vi "Mindsensors TouchMux Config.vi"(10 "Node Data":T1, 11 "NXT":T2) -> ()   [LabVIEW 2010]
uses:
  <vilib>/NXT/Subs/LVHSConnector.ctl
  Datatypes/Node.ctl
  UI Controls/PlugInControls/Pluginbackground.ctl
  <vilib>/Utility/miscctls.llb/LVPointTypeDef.ctl
  <vilib>/NXT/Block Support/HWPage.SensorType.ctl
  <vilib>/NXT/Block Support/HWPage.SensorMode.ctl
  ConvertNodeAddrSensor.vi
panel:
  out "TouchMux 3":bool
  out "TouchMux 2":bool
  out "TouchMux 1":bool
  in  "Output":string
  out "?":dbl format="%#.2g"
  out "number":i8
  in  "NXT Port":string
  in  "Name":string
  out "Headline":string="Type (auto populated)"
  in  "Sensor Parameters":string
  in  "Instance Specific Data":cluster{"Example Data":dbl}
  in  "Reset":bool
  in  "Save":bool
  in  "Stop":bool
  out "Background":T3=TRUE
  # "<- No controls below this line"
  # "Common controls such as Buttons, Rings, Sliders, Graphs, Decorations, etc can be found in the <labview>\\Targets\\NI\\NXT\\NXT Toolkit\\Schematic Editor\\UI Controls\\Plugin Controls\\ folder. Use these controls when possible to ensure a consistent look and feel with LabVIEW Education Edition."
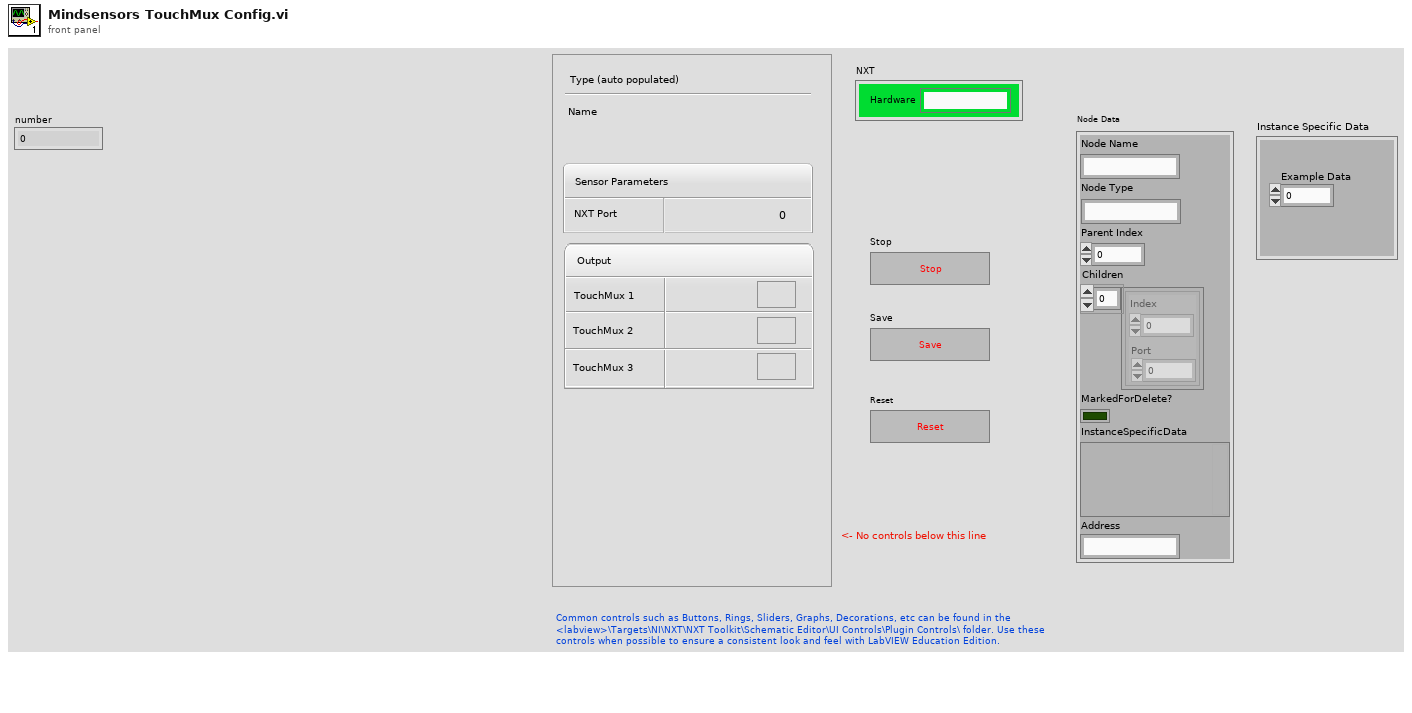
[diagram p1: front panel]
types:
  T1 = typedef "Node.ctl" = cluster{"Node Name":string, "Node Type":string, "Parent Index":i16, "Children":cluster{"Index":u16, "Port":u16}[], "MarkedForDelete?":bool, "InstanceSpecificData":variant, "Address":string}
  T2 = typedef "LVHSConnector.ctl" = cluster{"Hardware":string, "Flattened String":string}
  T3 = typedef "Pluginbackground.ctl" = bool
  T4 = typedef "LVPointTypeDef.ctl" = cluster{"Horizontal":i16, "Vertical":i16}
  T5 = typedef "HWPage.SensorType.ctl" = u8
  T6 = typedef "HWPage.SensorMode.ctl" = u8
  T7 = enum8{"Enabled", "Disabled", "Disabled and Grayed Out"}
  T8 = typedef "NXT_InputPort.ctl" = u8
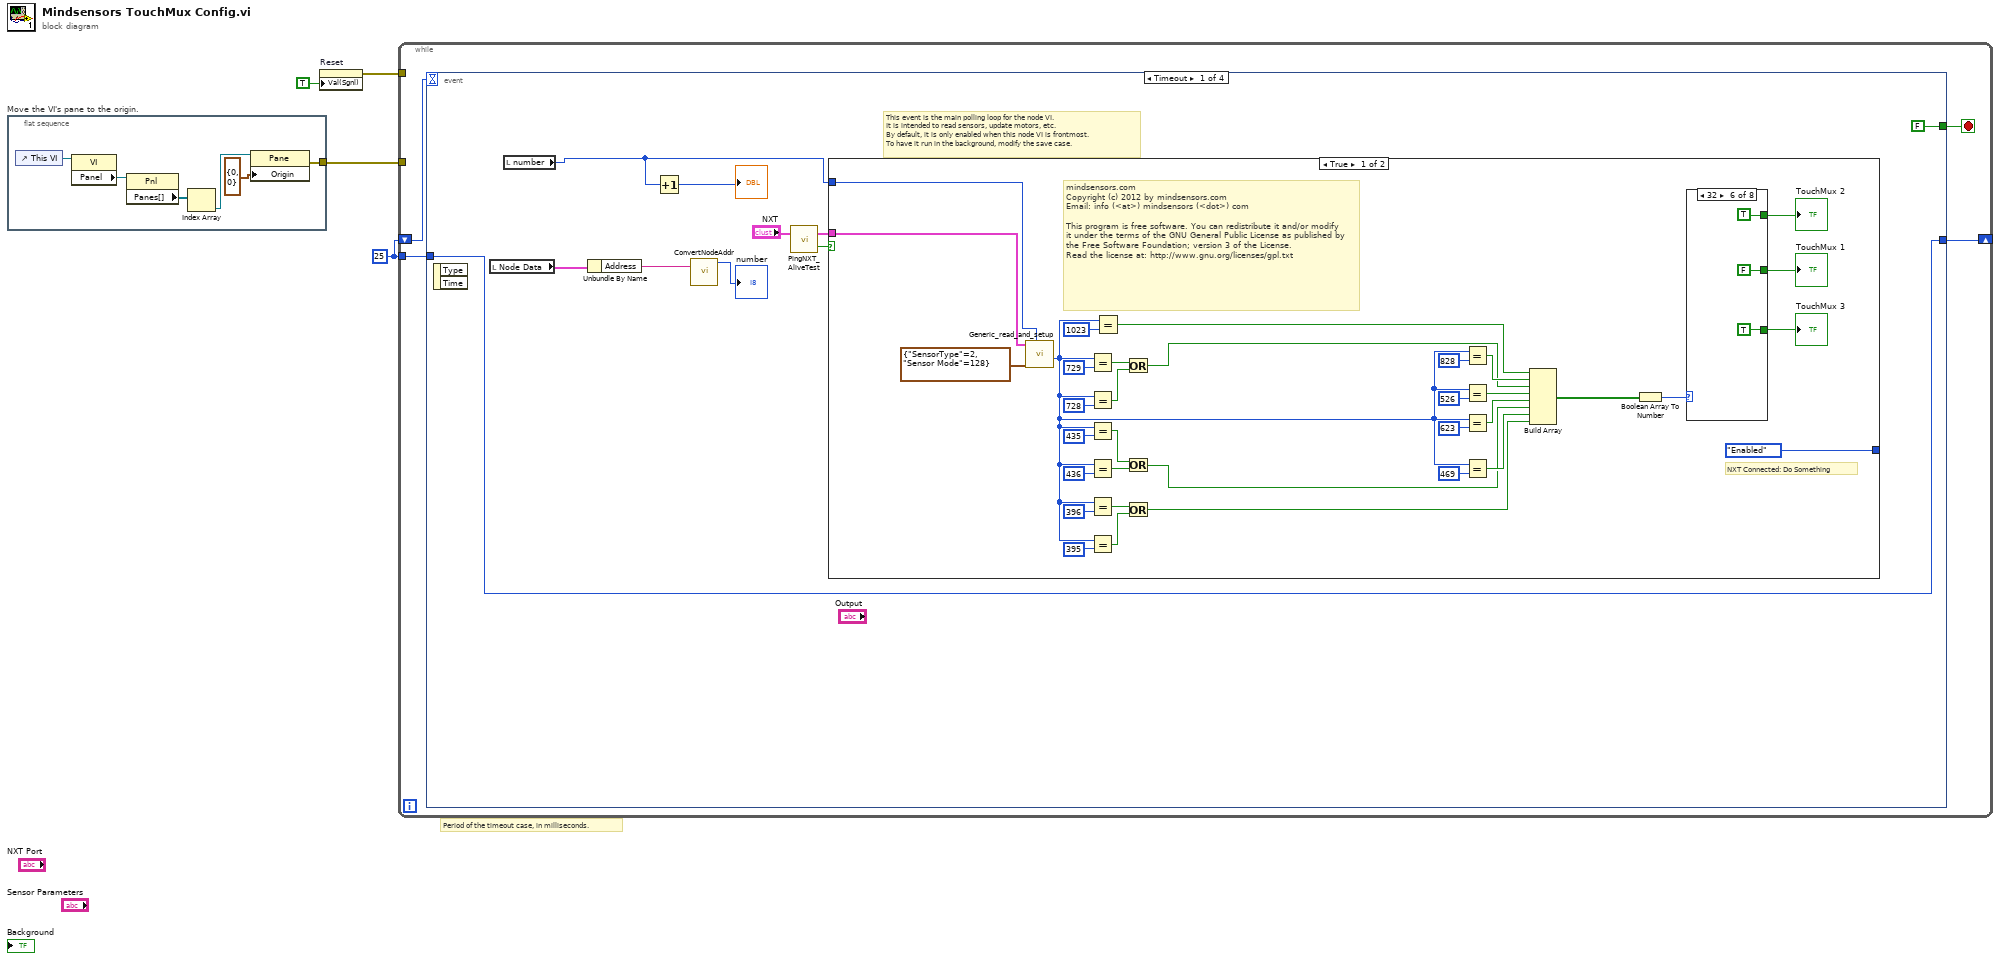
[diagram p0: block diagram]
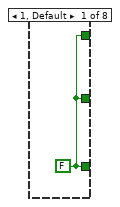
[diagram p2: hidden frame]
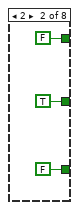
[diagram p3: hidden frame]
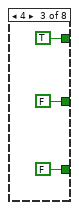
[diagram p4: hidden frame]
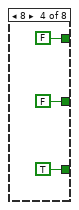
[diagram p5: hidden frame]
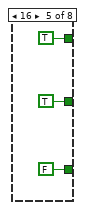
[diagram p6: hidden frame]
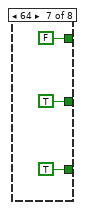
[diagram p7: hidden frame]
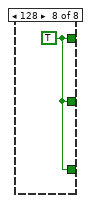
[diagram p8: hidden frame]
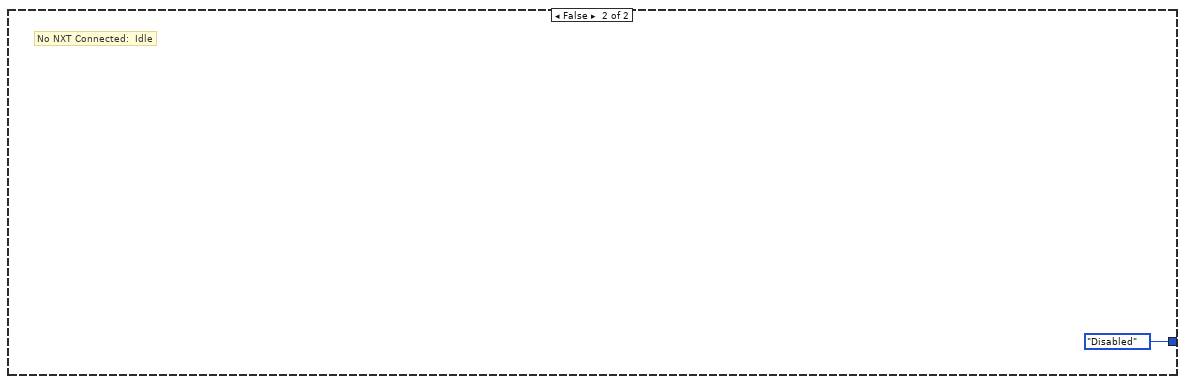
[diagram p9: hidden frame]
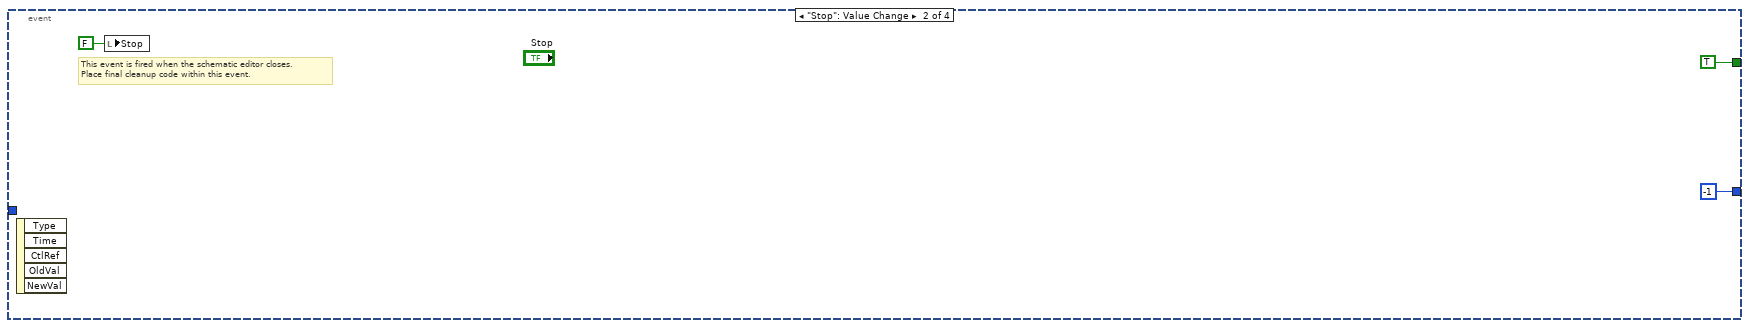
[diagram p10: hidden frame]
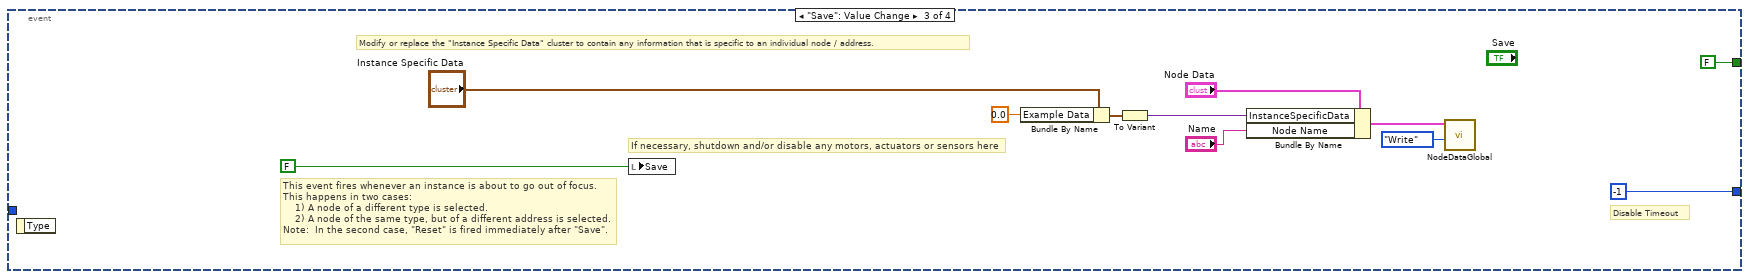
[diagram p11: hidden frame]
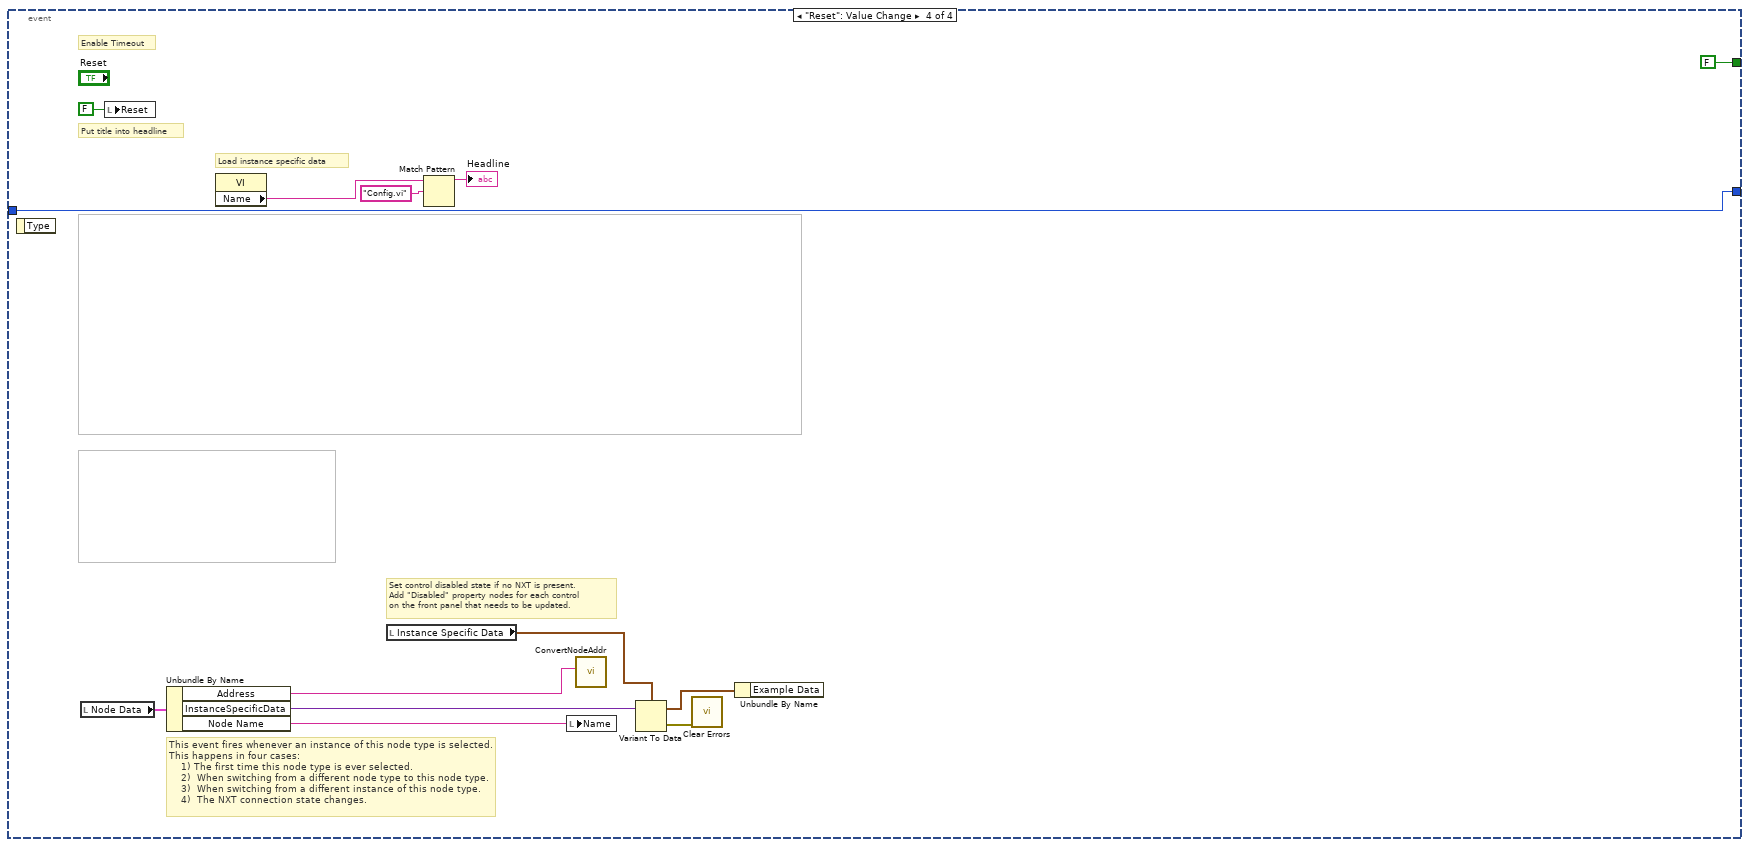
[diagram p12: hidden frame]
diagram:
  w2 = 25
  # "Period of the timeout case, in milliseconds."
  n1 = flat-sequence "Move the VI's pane to the origin." {
    tunnel: [w5] -> w1
    frame #0 {
      n2 = control-ref of="This VI"() -> (w6:refnum<vi>)
      n3 = property class="VI"(reference=w6) -> ("Panel"=w7:refnum<vi>)  [unwired: 1 in, 2 out]
      n4 = property class="Pnl"(reference=w7) -> ("Panes[]"=w8:refnum<vi>[])  [unwired: 1 in, 2 out]
      n5 = Index Array(array=w8) -> (element=w9:refnum<vi>)  [unwired: 1 in]
      n6 = property class="Pane"(reference=w9, "Origin"=T4 {"Horizontal"=0, "Vertical"=0}) -> (error out=w5:errorcluster)  [unwired: 1 in, 1 out]
    }
  }
  n7 = property on="Reset" class="Bool (strict)"("Val(Sgnl)"=TRUE ("Value (Signaling)")) -> (error out=w3:errorcluster)  [unwired: 2 in, 1 out]
  n8 = while {
    tunnel: w3 -> [_]
    shift-right: [w12] -> _
    shift-left: w2 -> [w13]
    tunnel: w2 -> [w11]
    tunnel: w1 -> [_]
    stop <- w14 stop-if-true
    n9 = event shown="[0] Timeout" {
      selector: _ -> [_ _ _ _]
      dyn-events: _ -> [_ _ _ _]
      timeout: w13 -> [_ _ _ _]
      tunnel: [FALSE TRUE FALSE FALSE] -> w14
      tunnel: [w23 -1 -1 w103] -> w12
      tunnel: w11 -> [w23 _ _ w103]
      event Timeout {
        # "This event is the main polling loop for the node VI.\nIt is intended to read sensors, update motors, etc.\nBy default, it is only enabled when this node VI is frontmost.\nTo have it run in the background, modify the save case."
        n10 = event-data() -> ()  [unwired: 1 in, 2 out]
        n11 = local read "Node Data"() -> (w21:T1)
        n12 = local read "number"() -> (w16:i8)
        n13 = Unbundle By Name(w21) -> ("Address"=w18:string)
        n14 = Increment(x=w16) -> (x+1=→"?":i8)
        n15 = call-poly "ConvertNodeAddr.vi"("Sensor Port"=w18) -> ("NXT Port"=→"number":T8)  [unwired: 6 in, 4 out]
        n16 = call <vilib>:"PingNXT_AliveTest.vi"("NXT"="NXT") -> ("connected?"=w20:bool, "NXT"=w19:T2)  [unwired: 1 in]
        n17 = case shown="True" w20 {
          tunnel: [T7."Enabled" ("Disabled") T7."Disabled" ("Disabled")] -> _
          tunnel: w19 -> [w57 _]
          tunnel: w16 -> [w58 _]
          frame True {
            # "mindsensors.com\nCopyright (c) 2012 by mindsensors.com\nEmail: info (<at>) mindsensors (<dot>) com\n\nThis program is free software. You can redistribute it and/or modify\nit under the terms of the GNU General Public License as published by\nthe Free Software Foundation; version 3 of the License.\nRead the license at: http://www.gnu.org/licenses/gpl.txt"
            # "NXT Connected: Do Something"
            n18 = call <vilib>:"Generic_read_and_setup.vi"("Port"=w58, "Sensor Setup"=cluster{"SensorType":T5, "Sensor Mode":T6} {"SensorType"=2, "Sensor Mode"=128}, "NXT In"=w57) -> ("Raw"=w28:u16)  [unwired: 6 in, 2 out]
            n19 = Equal?(x=w28, y=u16 729) -> (x = y?=w37:bool)
            n20 = Equal?(x=w28, y=u16 728) -> (x = y?=w35:bool)
            n21 = Equal?(x=w28, y=u16 435) -> (x = y?=w32:bool)
            n22 = Equal?(x=w28, y=u16 436) -> (x = y?=w31:bool)
            n23 = Equal?(x=w28, y=u16 396) -> (x = y?=w26:bool)
            n24 = Equal?(x=w28, y=u16 395) -> (x = y?=w27:bool)
            n25 = Equal?(x=w28, y=1023) -> (x = y?=w52:bool)
            n26 = Or(x=w37, y=w35) -> (x .or. y?=w34:bool)
            n27 = Or(x=w32, y=w31) -> (x .or. y?=w30:bool)
            n28 = Or(x=w26, y=w27) -> (x .or. y?=w25:bool)
            n29 = Equal?(x=w28, y=u16 828) -> (x = y?=w51:bool)
            n30 = Equal?(x=w28, y=u16 526) -> (x = y?=w50:bool)
            n31 = Equal?(x=w28, y=u16 623) -> (x = y?=w42:bool)
            n32 = Equal?(x=w28, y=u16 469) -> (x = y?=w41:bool)
            n33 = Build Array(w52, w51, w34, w50, w42, w30, w41, w25) -> (w55:bool[])
            n34 = Boolean Array To Number(Boolean array=w55) -> (number=w54:u32)
            n35 = case shown="32" w54 {
              tunnel: [w60 FALSE ("TouchMux 3") FALSE ("TouchMux 3") TRUE ("TouchMux 3") FALSE ("TouchMux 3") TRUE ("TouchMux 3") TRUE ("TouchMux 3") w79] -> w40
              tunnel: [w60 FALSE ("TouchMux 3") TRUE ("TouchMux 3") FALSE ("TouchMux 3") TRUE ("TouchMux 3") TRUE ("TouchMux 3") FALSE ("TouchMux 3") w79] -> w39
              tunnel: [w60 TRUE ("TouchMux 3") FALSE ("TouchMux 3") FALSE ("TouchMux 3") TRUE ("TouchMux 3") FALSE ("TouchMux 3") TRUE ("TouchMux 3") w79] -> w38
              frame 1, Default {
                w60 = FALSE ("TouchMux 3")
              }
              frame 2 {
              }
              frame 4 {
              }
              frame 8 {
              }
              frame 16 {
              }
              frame 32 {
              }
              frame 64 {
              }
              frame 128 {
                w79 = TRUE ("TouchMux 3")
              }
            }
            "TouchMux 1" <- w38
            "TouchMux 2" <- w39
            "TouchMux 3" <- w40
          }
          frame False {
            # "No NXT Connected:  Idle"
          }
        }
      }
      event "Stop": Value Change {
        # "This event is fired when the schematic editor closes.\nPlace final cleanup code within this event."
        n36 = event-data() -> ()  [unwired: 1 in, 5 out]
        n37 = local write "Stop"(FALSE ("stop")) -> ()
      }
      event "Save": Value Change {
        # "If necessary, shutdown and/or disable any motors, actuators or sensors here"
        # "Modify or replace the \"Instance Specific Data\" cluster to contain any information that is specific to an individual node / address."
        # "Disable Timeout"
        # "This event fires whenever an instance is about to go out of focus.\nThis happens in two cases:\n    1) A node of a different type is selected.\n    2) A node of the same type, but of a different address is selected.\nNote:  In the second case, \"Reset\" is fired immediately after \"Save\"."
        n38 = event-data() -> ()  [unwired: 1 in, 1 out]
        n39 = local write "Save"(FALSE ("stop")) -> ()
        n40 = Bundle By Name(cluster="Instance Specific Data", "Example Data"=0.0) -> (w85:cluster{"Example Data":dbl})
        n41 = To Variant(anything=w85) -> (Variant=w92:variant)
        n42 = Bundle By Name(cluster="Node Data", "InstanceSpecificData"=w92, "Node Name"="Name") -> (w91:T1)
        n43 = call "NodeDataGlobal.vi"("Action"=enum16{"Read", "Write"}."Write", "Node Data In"=w91) -> ()  [unwired: 8 in, 2 out]
      }
      event "Reset": Value Change {
        # "Set control disabled state if no NXT is present.\nAdd \"Disabled\" property nodes for each control\non the front panel that needs to be updated."
        # "Load instance specific data"
        # "Enable Timeout"
        # "This event fires whenever an instance of this node type is selected.\nThis happens in four cases:\n    1) The first time this node type is ever selected.\n    2)  When switching from a different node type to this node type.\n    3)  When switching from a different instance of this node type. \n    4)  The NXT connection state changes."
        # "Put title into headline"
        n44 = event-data() -> ()  [unwired: 1 in, 1 out]
        n45 = local read "Node Data"() -> (w104:T1)
        n46 = local write "Reset"(FALSE ("Reset")) -> ()
        n47 = Unbundle By Name(w104) -> ("Address"=w95:string, "InstanceSpecificData"=w105:variant, "Node Name"=w97:string)
        n48 = property class="VI"() -> ("Name"=w99:string)  [unwired: 2 in, 2 out]
        n49 = local read "Instance Specific Data"() -> (w102:cluster{"Example Data":dbl})
        n50 = Match Pattern(string=w99, regular expression="Config.vi") -> (before substring=→"Headline":string)  [unwired: 1 in, 3 out]
        n51 = local write "Name"(w97) -> ()
        n52 = call-poly "ConvertNodeAddr.vi"("Sensor Port"=w95) -> ()  [unwired: 6 in, 5 out]
        n53 = Variant To Data(Variant=w105, type=w102) -> (error out=w101:errorcluster, data=w96:cluster{"Example Data":dbl})  [unwired: 1 in]
        n54 = call <vilib>:"Clear Errors.vi"("error in (no error)"=w101) -> ()  [unwired: 6 in, 1 out]
        n55 = Unbundle By Name(w96) -> ()  [unwired: 1 out]
      }
    }
  }
